vi "Database Recordset Get Column Properties.vi"(8 "error in (no error)":errorcluster caption="错误输入（无错误）", 9 "Index":i32, 11 "Database Recordset 输入":refnum<class "Database Recordset.lvclass"> caption="DNL_LabVIEW Object in") -> (0 "error out":errorcluster caption="错误输出", 1 "column properties":T1 {"Type" items=["adEmpty"=0, "adTinyInt"=16, "adSmallInt"=2, "adInteger"=3, "adBigInt"=20, "adUnsignedTinyInt"=17, "adUnsignedSmallInt"=18, "adUnsignedInt"=19, "adUnsignedBigInt"=21, "adSingle"=4, "adDouble"=5, "adCurrency"=6, "adDecimal"=14, "adNumeric"=131, "adBoolean"=11, "adError"=10, "adUserDefined"=132, "adVariant"=12, "adIDispatch"=9, "adIUnknown"=13, "adGUID"=72, "adDate"=7, "adDBDate"=133, "adDBTime"=134, "adDBTimeStamp"=135, "adBSTR"=8, "adChar"=129, "adVarChar"=200, "adLongVarChar"=201, "adWChar"=130, "adVarWChar"=202, "adLongVarWChar"=203, "adBinary"=128, "adVarBinary"=204, "adLongVarBinary"=205, "adChapter"=136, "adFileTime"=64, "adPropVariant"=138, "adVarNumeric"=139, "adArray"=8192]}, 3 "Database Recordset 输出":refnum<class "Database Recordset.lvclass"> caption="DNL_LabVIEW Object out")   [LabVIEW 2011, in "Database Recordset.lvclass"]
uses:
  Database Recordset.lvclass
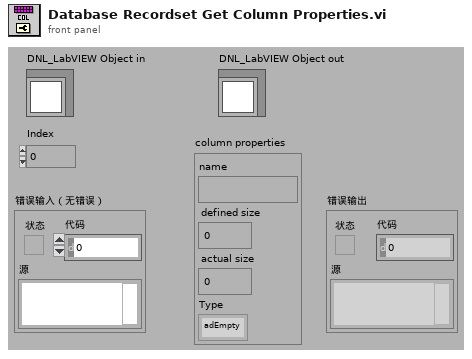
[diagram p1: front panel]
types:
  T1 = cluster{"name":string, "defined size":i32, "actual size":i32, "Type":i32}
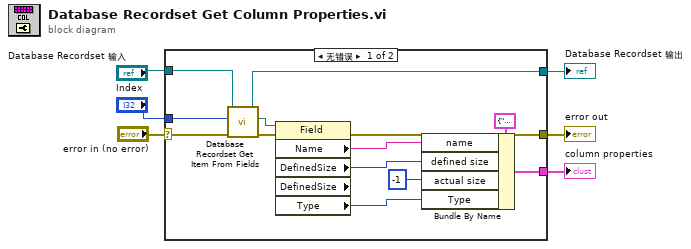
[diagram p0: block diagram]
diagram:
  n1 = case shown="无错误" "error in (no error)" {
    selector: "error in (no error)" -> [w8 w21]
    tunnel: [w10 w21] -> w5
    tunnel: [w14 w20] -> w3
    tunnel: "Database Recordset 输入" -> [w9 w20]
    tunnel: [w15 _] -> w2
    tunnel: "Index" -> [w11 _]
    frame No Error {
      n2 = call "Database Recordset Get Item From Fields.vi"("error in (no error)"=w8, "Index"=w11, "Database Recordset 输入"=w9) -> ("error out"=w13:errorcluster, "Item"=w12:refnum<k7>, "Database Recordset 输出"=w14:refnum<class "Database Recordset.lvclass">)  [unwired: 6 in]
      n3 = property class="Field" props=["Name", "DefinedSize", "DefinedSize", "Type"](reference=w12, error in=w13) -> (error out=w10:errorcluster, "Name"=w18:string, "DefinedSize"=w17:i32, "Type"=w16:i32)  [unwired: 2 out]
      n4 = Bundle By Name(cluster=T1 {"name"="", "defined size"=0, "actual size"=0, "Type"=0} ("column properties"), "name"=w18, "defined size"=w17, "actual size"=-1, "Type"=w16) -> (w15:T1)
    }
    frame Error {
    }
  }
  "error out" <- w5
  "Database Recordset 输出" <- w3
  "column properties" <- w2
